vi "Power Peak Calibration Inputs to XML.vi"() -> (0 "XML Data":string)   [LabVIEW 2013]
uses:
  Types/Power Peak Calibration Inputs.ctl
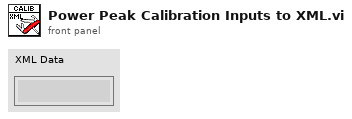
[diagram p1: front panel]
types:
  T1 = typedef "Power Peak Calibration Inputs.ctl" = cluster{"Number of Sweeps":dbl, "Calibration Sample Rate":dbl, "Samples Per Sweep":dbl, "Version":string}
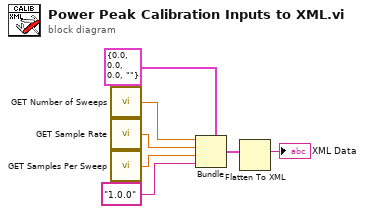
[diagram p0: block diagram]
diagram:
  n1 = call "GET Number of Sweeps.vi"() -> ("Number of Sweeps"=w3:dbl)
  n2 = call "GET Sample Rate.vi"() -> ("Calibration Sample Rate"=w5:dbl)
  n3 = call "GET Samples Per Sweep.vi"() -> ("Samples Per Sweep"=w6:dbl)
  n4 = Bundle(cluster=T1 {"Number of Sweeps"=0.0, "Calibration Sample Rate"=0.0, "Samples Per Sweep"=0.0, "Version"=""} ("Power Peak Calibration Inputs"), "Number of Sweeps"=w3, "Calibration Sample Rate"=w5, "Samples Per Sweep"=w6, "Version"="1.0.0") -> (w7:T1)
  n5 = Flatten To XML(anything=w7) -> (xml string=→"XML Data":string)
